vi "resolveAxisLetter.vi"(8 "error in (no error)":errorcluster, 10 "Axis Letter in":string, 11 "Controller in":refnum<class "Controller.lvclass">) -> (0 "error out":errorcluster, 2 "Axis Letter out":string, 3 "Controller out":refnum<class "Controller.lvclass">)   [LabVIEW 2019, in "Controller.lvclass"]
uses:
  Controller.lvclass
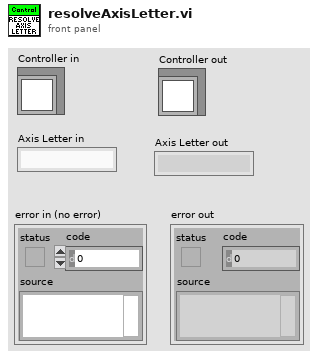
[diagram p1: front panel]
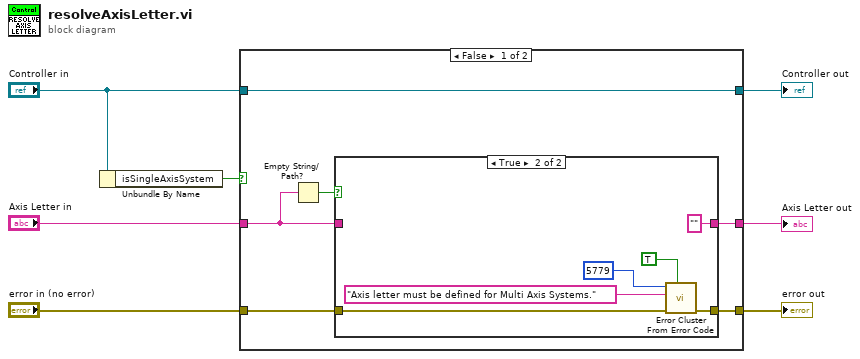
[diagram p0: block diagram]
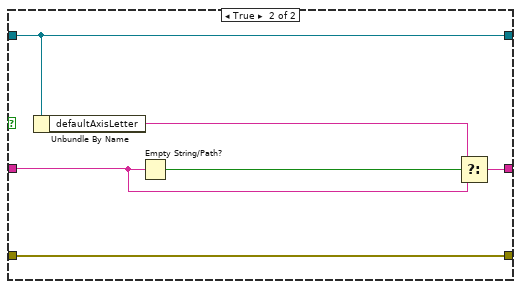
[diagram p3: hidden frame]
diagram:
  n1 = Unbundle By Name("Controller in") -> ("isSingleAxisSystem"=w5:bool)
  n2 = case shown="False" w5 {
    tunnel: [w10 w26] -> w7
    tunnel: "Axis Letter in" -> [w9 w25]
    tunnel: [w11 w23] -> w4
    tunnel: "error in (no error)" -> [w12 w23]
    tunnel: "Controller in" -> [w13 w22]
    tunnel: [w13 w22] -> w1
    frame False {
      n3 = Empty String/Path?(string/path=w9) -> (empty?=w8:bool)
      n4 = case shown="True" w8 {
        tunnel: w12 -> [w15 w20]
        tunnel: [w15 w19] -> w11
        tunnel: [w14 "" ("Axis Letter in")] -> w10
        tunnel: w9 -> [w14 _]
        frame False {
        }
        frame True {
          n5 = call <vilib>:"Error Cluster From Error Code.vi"("show call chain? (False)"=TRUE, "error in (no error)"=w20, "error message (\"\")"="Axis letter must be defined for Multi Axis Systems." ("error message (\"\")"), "error code (0)"=5779) -> ("error out"=w19:errorcluster)  [unwired: 5 in]
        }
      }
    }
    frame True {
      n6 = Unbundle By Name(w22) -> ("defaultAxisLetter"=w27:string)
      n7 = Empty String/Path?(string/path=w25) -> (empty?=w24:bool)
      n8 = Select(t=w27, s=w24, f=w25) -> (s? t:f=w26:string)
    }
  }
  "Axis Letter out" <- w7
  "Controller out" <- w1
  "error out" <- w4
